vi "Flat.vi"() -> ()   [LabVIEW 2020]
uses:
  <instrlib>/niDMM/nidmm.llb/niDMM Function.ctl
  <instrlib>/niDMM/nidmm.llb/niDMM Resolution in Digits.ctl
  <instrlib>/niDCPower/nidcpower.llb/niDCPower Output Function.ctl
  <instrlib>/niDCPower/nidcpower.llb/niDCPower Source Mode.ctl
  <instrlib>/niDMM/nidmm.llb/niDMM Configure Measurement Digits.vi
panel:
  in  "Load Current":dbl=0.1 format="%#_13p"
  in  "SMU Load":refnum<k15>="SMU_Load"
  in  "SMU Source":refnum<k15>="SMU_Source"
  in  "DMM2":refnum<k15>="Measure_Load"
  in  "DMM1":refnum<k15>="Measure_Source"
  in  "Required Drop in Vout (V)":dbl=0.1 format="%_1p"
  in  "Nominal Voltage (V)":dbl=4.88 format="%_4p"
  in  "SMU Voltage Scan Parameters":T1={"Vin Start Voltage (V)"=6.5, "Vin Stop Voltage Level (V)"=4.0, "Voltage Step (V)"=0.1} {"Vin Start Voltage (V)" format="%#_13g"}
  out "Dropout Voltage (V)":dbl format="%#_3p"
  out "LDO Vout vs Vin Graph":cluster{dbl[], dbl[]}(graph)={[50.00221359436212, 50.000632455532035, 50.000632455532035, 50.00284604989415, 50.00284604989415, 50.000632455532035, 50.000632455532035, 50.00094868329805, 50.00094868329805, 50.0, 50.0, 50.00158113883008, 50.00158113883008, 50.00126491106407, 50.00126491106407, 50.000316227766014, 50.000316227766014, 50.0, 50.0, 50.00284604989415, 50.00284604989415, 50.00094868329805, 50.00094868329805, 50.00252982212813, 50.00252982212813, 50.000316227766014], [50.00221359436212, 50.000632455532035, 50.000632455532035, 50.00284604989415, 50.00284604989415, 50.000632455532035, 50.000632455532035, 50.00094868329805, 50.00094868329805, 50.0, 50.0, 50.00158113883008, 50.00158113883008, 50.00126491106407, 50.00126491106407, 50.000316227766014, 50.000316227766014, 50.0, 50.0, 50.00284604989415, 50.00284604989415, 50.00094868329805, 50.00094868329805, 50.00252982212813, 50.00252982212813, 50.000316227766014]}
  in  "stop":bool
  out "[Vout_nom - Vout_req.Drop] (V)":dbl
  out "Vin(V) @ [Vout_nom - Vout_req.Drop] (V)":dbl
  out "Measurement Results\n(Vin, Vout)":dbl[][](array[numeric]) format="%_5p"
  # "LDO Dropout Voltage Measurement"
  # "LDO Dropout Voltage Measurement"
  # "Test Results"
  # "Debug"
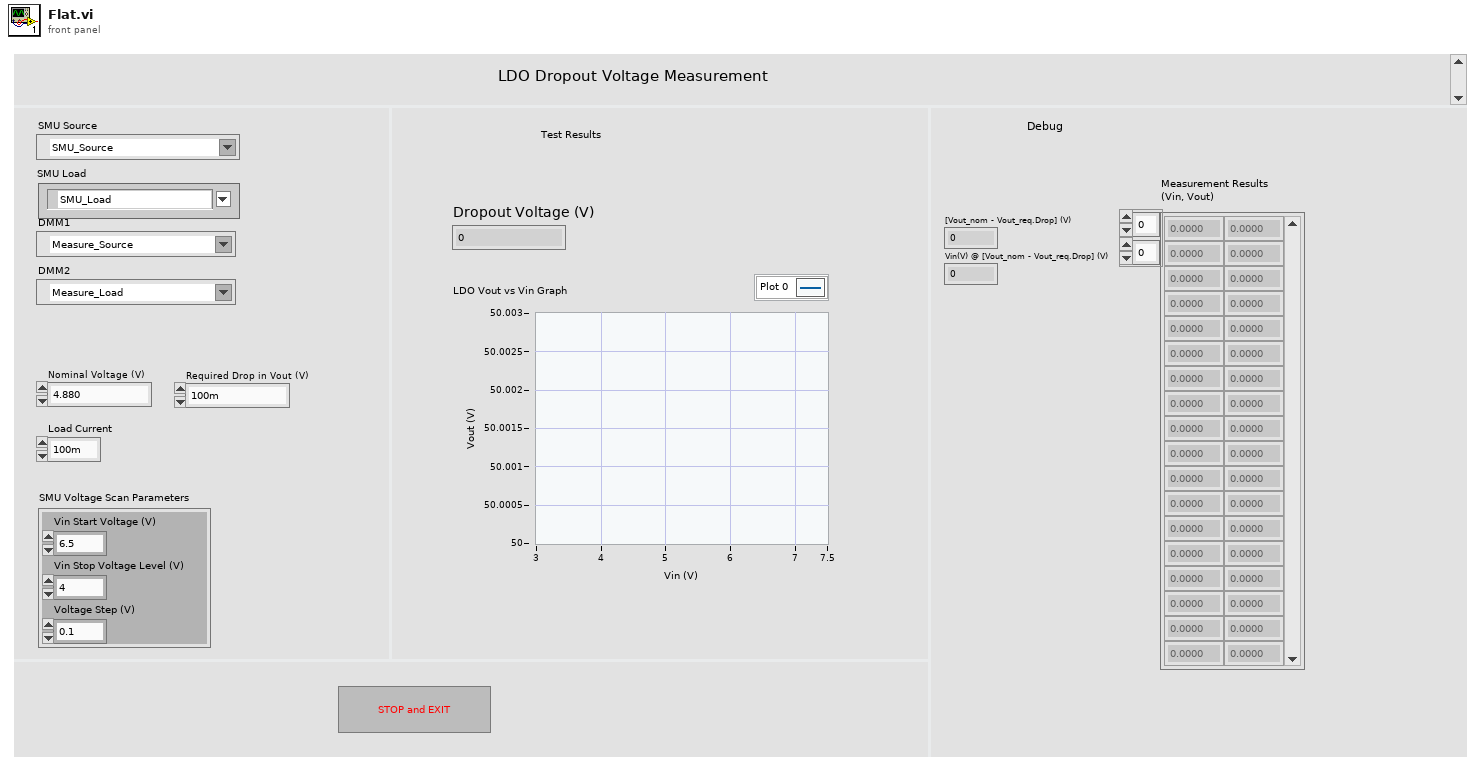
[diagram p1: front panel]
types:
  T1 = cluster{"Vin Start Voltage (V)":dbl, "Vin Stop Voltage Level (V)":dbl, "Voltage Step (V)":dbl}
  T2 = typedef "niDCPower Output Function.ctl" = i32
  T3 = typedef "niDCPower Source Mode.ctl" = i32
  T4 = typedef "niDMM Resolution in Digits.ctl" = dbl
  T5 = typedef "niDMM Function.ctl" = enum16{"DC Volts", "AC Volts", "DC Current", "AC Current", "2-wire Resistance", "4-wire Resistance", "Diode", "Frequency", "Period", "AC Volts DC Coupled", "Capacitance", "Inductance", "Temperature"}
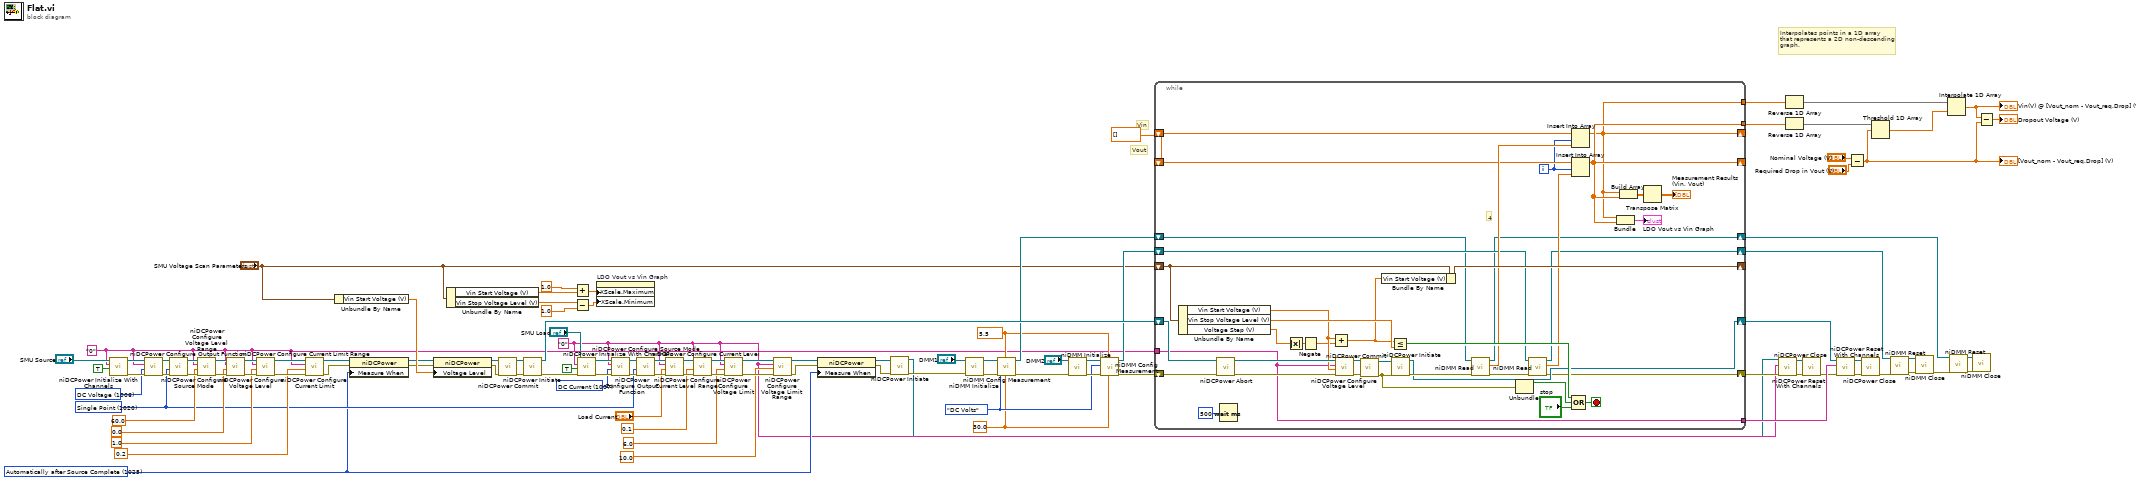
[diagram p0: block diagram]
diagram:
  w23 = T2 1007 items=["DC Voltage"=1006, "DC Current"=1007, "Pulse Voltage"=1049, "Pulse Current"=1050] ("output function")
  w2 = "0" ("channel")
  w25 = T3 1020 items=["Single Point"=1020, "Sequence"=1021] ("source mode")
  w47 = "0" ("channel")
  w46 = T2 1006 items=["DC Voltage"=1006, "DC Current"=1007, "Pulse Voltage"=1049, "Pulse Current"=1050] ("output function")
  w50 = 30.0 ("Range")
  w49 = T4 5.5 items=["3 1/2"=3.5, "4 1/2"=4.5, "5 1/2"=5.5, "6 1/2"=6.5, "7 1/2"=7.5] ("Resolution in Digits")
  w51 = niDMM_Function."DC Volts" ("Function")
  w71 = dbl[] []
  w18 = 1025 items=["Automatically after Source Complete"=1025, "On Demand"=1026, "On Measure Trigger"=1027] ("Measurement:Advanced:Measure When")
  # "Interpolates points in a 1D array \nthat represents a 2D non-descending \ngraph."
  # "Vout"
  # "Vin"
  n1 = call <instrlib>:"niDCPower Initialize With Channels.vi"("reset (false)"=TRUE, "channels"=w47, "resource name"="SMU Source") -> ("error out"=w92:errorcluster, "instrument handle out"=w93:refnum<k15>)  [unwired: 7 in]
  n2 = call <instrlib>:"niDCPower Configure Output Function.vi"("error in (no error)"=w92, "output function"=w46, "channel name"=w47, "instrument handle"=w93) -> ("error out"=w105:errorcluster, "instrument handle out"=w106:refnum<k15>)  [unwired: 6 in]
  n3 = call <instrlib>:"niDCPower Configure Source Mode.vi"("error in (no error)"=w105, "source mode"=w25, "instrument handle"=w106) -> ("error out"=w100:errorcluster, "instrument handle out"=w104:refnum<k15>)  [unwired: 7 in]
  n4 = call <instrlib>:"niDCPower Configure Voltage Level Range.vi"("error in (no error)"=w100, "voltage level range"=60.0, "channel name"=w47, "instrument handle"=w104) -> ("error out"=w99:errorcluster, "instrument handle out"=w103:refnum<k15>)  [unwired: 6 in]
  n5 = call <instrlib>:"niDCPower Configure Voltage Level.vi"("error in (no error)"=w99, "voltage level"=0.0, "channel name"=w47, "instrument handle"=w103) -> ("error out"=w98:errorcluster, "instrument handle out"=w102:refnum<k15>)  [unwired: 6 in]
  n6 = call <instrlib>:"niDCPower Configure Current Limit Range.vi"("error in (no error)"=w98, "current limit range"=1.0, "channel name"=w47, "instrument handle"=w102) -> ("error out"=w97:errorcluster, "instrument handle out"=w101:refnum<k15>)  [unwired: 6 in]
  n7 = call <instrlib>:"niDCPower Configure Current Limit.vi"("error in (no error)"=w97, "current limit"=0.2, "channel name"=w47, "instrument handle"=w101) -> ("error out"=w81:errorcluster, "instrument handle out"=w85:refnum<k15>)  [unwired: 6 in]
  n8 = Unbundle By Name("SMU Voltage Scan Parameters") -> ("Vin Start Voltage (V)"=w86:dbl)
  n9 = property class="niDCPower"(reference=w85, error in=w81, "Measure When"=w18) -> (reference out=w84:refnum<k15>, error out=w83:errorcluster)
  n10 = property class="niDCPower"(reference=w84, error in=w83, "Voltage Level"=w86) -> (reference out=w91:refnum<k15>, error out=w94:errorcluster)
  n11 = Unbundle By Name("SMU Voltage Scan Parameters") -> ("Vin Start Voltage (V)"=w69:dbl, "Vin Stop Voltage Level (V)"=w65:dbl)
  n12 = call <instrlib>:"niDCPower Commit.vi"("error in (no error)"=w94, "instrument handle"=w91) -> ("error out"=w95:errorcluster, "instrument handle out"=w96:refnum<k15>)  [unwired: 8 in]
  n13 = call <instrlib>:"niDCPower Initiate.vi"("error in (no error)"=w95, "instrument handle"=w96) -> ("error out"=w40:errorcluster, "instrument handle out"=w82:refnum<k15>)  [unwired: 8 in]
  n14 = Add(x=1.0, y=w69) -> (x+y=w67:dbl)
  n15 = Subtract(x=w65, y=1.0 ("x")) -> (x-y=w66:dbl)
  n16 = call <instrlib>:"niDCPower Initialize With Channels.vi"("error in (no error)"=w40, "reset (false)"=TRUE, "channels"=w2, "resource name"="SMU Load") -> ("error out"=w26:errorcluster, "instrument handle out"=w24:refnum<k15>)  [unwired: 6 in]
  n17 = property on="LDO Vout vs Vin Graph" class="XYGraph (strict)"("XScale.Maximum"=w67, "XScale.Minimum"=w66) -> ()  [unwired: 2 in, 2 out]
  n18 = call <instrlib>:"niDCPower Configure Output Function.vi"("error in (no error)"=w26, "output function"=w23, "channel name"=w2, "instrument handle"=w24) -> ("error out"=w37:errorcluster, "instrument handle out"=w38:refnum<k15>)  [unwired: 6 in]
  n19 = call <instrlib>:"niDCPower Configure Source Mode.vi"("error in (no error)"=w37, "source mode"=w25, "instrument handle"=w38) -> ("error out"=w32:errorcluster, "instrument handle out"=w36:refnum<k15>)  [unwired: 7 in]
  n20 = call <instrlib>:"niDCPower Configure Current Level.vi"("error in (no error)"=w32, "current level"="Load Current", "channel name"=w2, "instrument handle"=w36) -> ("error out"=w31:errorcluster, "instrument handle out"=w35:refnum<k15>)  [unwired: 6 in]
  n21 = call <instrlib>:"niDCPower Configure Current Level Range.vi"("error in (no error)"=w31, "current level range"=0.1, "channel name"=w2, "instrument handle"=w35) -> ("error out"=w30:errorcluster, "instrument handle out"=w34:refnum<k15>)  [unwired: 6 in]
  n22 = call <instrlib>:"niDCPower Configure Voltage Limit.vi"("error in (no error)"=w30, "voltage limit"=6.0, "channel name"=w2, "instrument handle"=w34) -> ("error out"=w29:errorcluster, "instrument handle out"=w33:refnum<k15>)  [unwired: 6 in]
  n23 = call <instrlib>:"niDCPower Configure Voltage Limit Range.vi"("error in (no error)"=w29, "voltage limit range"=10.0, "channel name"=w2, "instrument handle"=w33) -> ("error out"=w27:errorcluster, "instrument handle out"=w28:refnum<k15>)  [unwired: 6 in]
  n24 = property class="niDCPower"(reference=w28, error in=w27, "Measure When"=w18) -> (reference out=w15:refnum<k15>, error out=w17:errorcluster)
  n25 = call <instrlib>:"niDCPower Initiate.vi"("error in (no error)"=w17, "instrument handle"=w15) -> ("error out"=w16:errorcluster, "instrument handle out"=w1:refnum<k15>)  [unwired: 8 in]
  n26 = call <instrlib>:"niDMM Initialize.vi"("error in (no error)"=w16, "Instrument Descriptor"="DMM1") -> ("error out"=w79:errorcluster, "instrument handle out"=w80:refnum<k15>)  [unwired: 8 in]
  n27 = call-poly <instrlib>:"niDMM Config Measurement.vi"("Range"=w50, "Resolution in Digits"=w49, "error in (no error)"=w79, "Function"=w51, "instrument handle"=w80) -> ("error out"=w77:errorcluster, "instrument handle out"=w78:refnum<k15>)  [unwired: 5 in]
  n28 = call <instrlib>:"niDMM Initialize.vi"("error in (no error)"=w77, "Instrument Descriptor"="DMM2") -> ("error out"=w74:errorcluster, "instrument handle out"=w73:refnum<k15>)  [unwired: 8 in]
  n29 = call-poly <instrlib>:"niDMM Config Measurement.vi"("Range"=w50, "Resolution in Digits"=w49, "error in (no error)"=w74, "Function"=w51, "instrument handle"=w73) -> ("error out"=w76:errorcluster, "instrument handle out"=w75:refnum<k15>)  [unwired: 5 in]
  n30 = while {
    shift-right: [w130] -> w89
    shift-left: w82 -> [w146]
    shift-right: [w119] -> w4
    shift-left: w76 -> [w145]
    shift-right: [w137] -> _
    shift-left: "SMU Voltage Scan Parameters" -> [w139]
    tunnel: w47 -> [w117]
    shift-right: [w120] -> w9
    shift-left: w75 -> [w122]
    shift-right: [w121] -> w7
    shift-left: w78 -> [w118]
    tunnel: [w117] -> w72
    shift-right: [w108] -> _
    shift-left: w71 -> [w116]
    shift-right: [w109] -> _
    shift-left: w71 -> [w115]
    tunnel: [w109] -> w63
    tunnel: [w108] -> w62
    i -> [w114]
    stop <- w136 stop-if-true
    # "4"
    n31 = Unbundle By Name(w139) -> ("Vin Start Voltage (V)"=w132:dbl, "Vin Stop Voltage Level (V)"=w140:dbl, "Voltage Step (V)"=w141:dbl)
    n32 = call <instrlib>:"niDCPower Abort.vi"("error in (no error)"=w145, "instrument handle"=w146) -> ("error out"=w143:errorcluster, "instrument handle out"=w144:refnum<k15>)  [unwired: 8 in]
    n33 = Wait (ms)(milliseconds to wait=u32 500) -> ()  [unwired: 1 out]
    n34 = Absolute Value(x=w141) -> (abs(x)=w110:dbl)
    n35 = Negate(x=w110) -> (-x=w107:dbl)
    n36 = Add(x=w132, y=w107) -> (x+y=w138:dbl)
    n37 = call <instrlib>:"niDCPower Configure Voltage Level.vi"("error in (no error)"=w143, "voltage level"=w132, "channel name"=w117, "instrument handle"=w144) -> ("error out"=w128:errorcluster, "instrument handle out"=w129:refnum<k15>)  [unwired: 6 in]
    n38 = call <instrlib>:"niDCPower Commit.vi"("error in (no error)"=w128, "instrument handle"=w129) -> ("error out"=w126:errorcluster, "instrument handle out"=w127:refnum<k15>)  [unwired: 8 in]
    n39 = Bundle By Name(cluster=w139, "Vin Start Voltage (V)"=w138) -> (w137:T1)
    n40 = Less Or Equal?(x=w138, y=w140) -> (x <= y?=w135:bool)
    n41 = call <instrlib>:"niDCPower Initiate.vi"("error in (no error)"=w126, "instrument handle"=w127) -> ("error out"=w131:errorcluster, "instrument handle out"=w130:refnum<k15>)  [unwired: 8 in]
    n42 = call <instrlib>:"niDMM Read.vi"("error in (no error)"=w131, "instrument handle"=w118) -> ("error out"=w124:errorcluster, "Measurement"=w125:dbl, "instrument handle out"=w121:refnum<k15>)  [unwired: 7 in]
    n43 = Unbundle(w126) -> ("status"=w134:bool)  [unwired: 2 out]
    n44 = call <instrlib>:"niDMM Read.vi"("error in (no error)"=w124, "instrument handle"=w122) -> ("error out"=w119:errorcluster, "Measurement"=w123:dbl, "instrument handle out"=w120:refnum<k15>)  [unwired: 7 in]
    n45 = Insert Into Array(array=w116, index=w114, new element=w125) -> (w108:dbl[])
    n46 = Insert Into Array(array=w115, index=w114, new element=w123) -> (w109:dbl[])
    n47 = Compound Arithmetic op=OR(w135, w134, "stop") -> (w136:bool)
    n48 = Bundle(w108, w109) -> (→"LDO Vout vs Vin Graph":cluster{dbl[], dbl[]})  [unwired: 1 in]
    n49 = Build Array(w108, w109) -> (w113:dbl[][])
    n50 = Transpose Matrix(1:w113) -> (0:→"Measurement Results\n(Vin, Vout)":dbl[][])
  }
  n51 = call <instrlib>:"niDCPower Reset With Channels.vi"("error in (no error)"=w4, "channel name"=w2, "instrument handle"=w1) -> ("error out"=w5:errorcluster, "instrument handle out"=w6:refnum<k15>)  [unwired: 7 in]
  n52 = Reverse 1D Array(array=w62) -> (reversed array=w58:dbl[])
  n53 = Reverse 1D Array(array=w63) -> (reversed array=w61:dbl[])
  n54 = call <instrlib>:"niDCPower Close.vi"("error in (no error)"=w5, "instrument handle"=w6) -> ("error out"=w3:errorcluster)  [unwired: 9 in]
  n55 = call <instrlib>:"niDCPower Reset With Channels.vi"("error in (no error)"=w3, "channel name"=w72, "instrument handle"=w89) -> ("error out"=w87:errorcluster, "instrument handle out"=w88:refnum<k15>)  [unwired: 7 in]
  n56 = Subtract(x="Nominal Voltage (V)", y="Required Drop in Vout (V)") -> (x-y=w55:dbl)
  "[Vout_nom - Vout_req.Drop] (V)" <- w55
  n57 = call <instrlib>:"niDCPower Close.vi"("error in (no error)"=w87, "instrument handle"=w88) -> ("error out"=w10:errorcluster)  [unwired: 9 in]
  n58 = Threshold 1D Array(2:w55, 3:w61) -> (0:w57:dbl)  [unwired: 1 in]
  n59 = call <instrlib>:"niDMM Reset.vi"("error in (no error)"=w10, "instrument handle"=w9) -> ("error out"=w14:errorcluster, "instrument handle out"=w8:refnum<k15>)  [unwired: 8 in]
  n60 = call <instrlib>:"niDMM Close.vi"("error in (no error)"=w14, "instrument handle"=w8) -> ("error out"=w11:errorcluster)  [unwired: 9 in]
  n61 = Interpolate 1D Array(1:w57, 2:w58) -> (0:w56:dbl)
  "Vin(V) @ [Vout_nom - Vout_req.Drop] (V)" <- w56
  n62 = call <instrlib>:"niDMM Reset.vi"("error in (no error)"=w11, "instrument handle"=w7) -> ("error out"=w13:errorcluster, "instrument handle out"=w12:refnum<k15>)  [unwired: 8 in]
  n63 = call <instrlib>:"niDMM Close.vi"("error in (no error)"=w13, "instrument handle"=w12) -> ()  [unwired: 9 in, 1 out]
  n64 = Subtract(x=w56, y=w55) -> (x-y=→"Dropout Voltage (V)":dbl)
